vi "数据主动和反控发送.vi"   [LabVIEW 2016, in "数据传输系统.lvlib"]
uses:
  <vilib>/ptbypt/NI_PtbyPt.lvlib
types:
  T1 = enum16{"00点", "01点", "02点", "03点", "04点", "05点", "06点", "07点", "08点", "09点", "10点", "11点", "12点", "13点", "14点", "15点", "16点", "17点", "18点", "19点", "20点", "21点", "22点", "23点"}
  T2 = enum16{"关闭", "星期日", "星期一", "星期二", "星期三", "星期四", "星期五", "星期六"}
  T3 = typedef "LVDateTimeRec.ctl" = cluster{"秒数的小数部分":dbl, "秒":i32, "分":i32, "时":i32, "日":i32, "月":i32, "年":i32, "天数（周）":i32, "天数（年）":i32, "DST":i32}
  T4 = cluster{"CODMn":bool, "CODCr":bool, "DO":bool, "铜":bool, "PH":bool, "氨氮":bool, "比电导率":bool, "水温":bool, "盐度(海水)":bool, "浊度":bool, "总氮":bool, "总磷":bool, "叶绿素a":bool, "藻密度":bool, "水位":bool, "流速":bool, "瞬时流量":bool, "累积流量":bool}
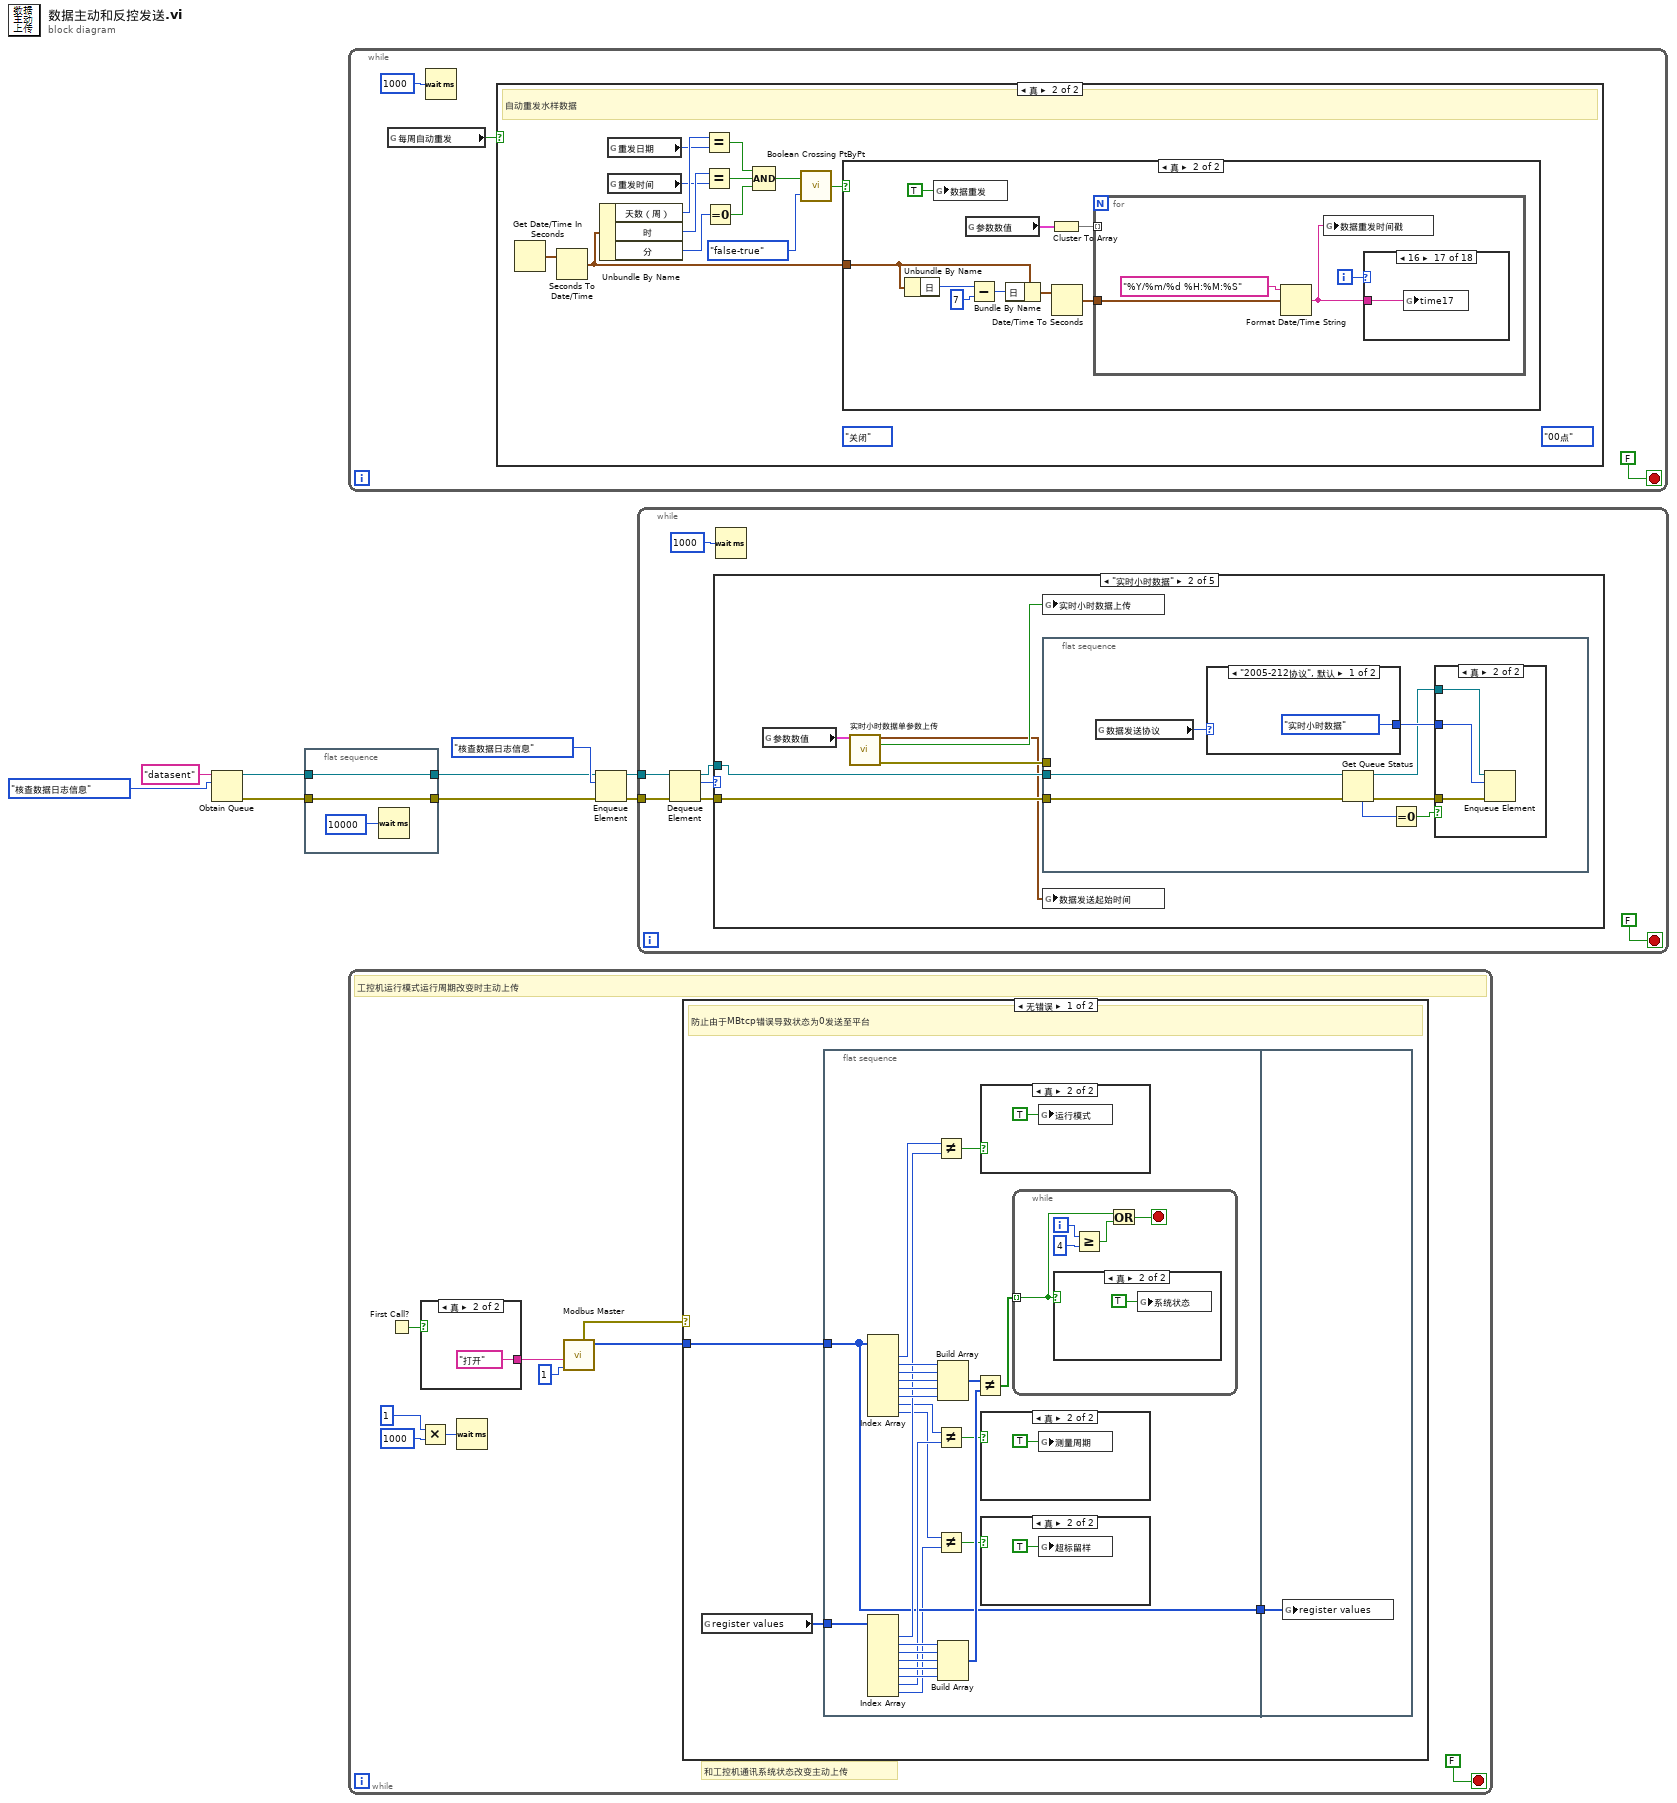
[diagram p0: block diagram]
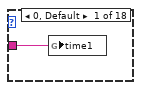
[diagram p4: hidden frame]
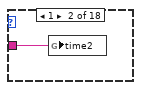
[diagram p5: hidden frame]
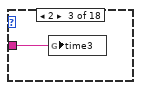
[diagram p6: hidden frame]
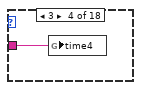
[diagram p7: hidden frame]
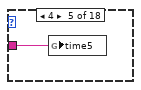
[diagram p8: hidden frame]
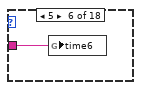
[diagram p9: hidden frame]
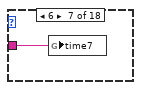
[diagram p10: hidden frame]
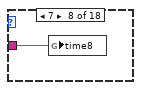
[diagram p11: hidden frame]
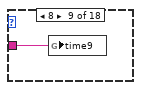
[diagram p12: hidden frame]
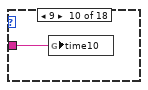
[diagram p13: hidden frame]
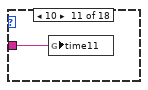
[diagram p14: hidden frame]
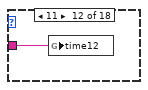
[diagram p15: hidden frame]
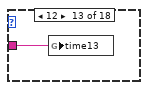
[diagram p16: hidden frame]
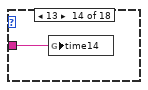
[diagram p17: hidden frame]
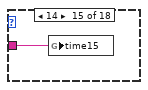
[diagram p18: hidden frame]
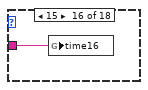
[diagram p19: hidden frame]
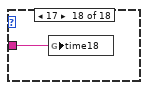
[diagram p20: hidden frame]
diagram:
  n1 = Obtain Queue(name (unnamed)="datasent" ("名称（未命名）"), element data type=enum16{"实时小时数据", "核查数据日志信息", "其他信息", "反控命令"}."核查数据日志信息") -> (queue out=w4:refnum<queue>, error out=w2:errorcluster)  [unwired: 3 in, 1 out]
  n2 = flat-sequence {
    tunnel: w4 -> [w11]
    tunnel: [w11] -> w3
    tunnel: w2 -> [w10]
    tunnel: [w10] -> w1
    frame #0 {
      n3 = Wait (ms)(milliseconds to wait=u32 10000 ("等待时间（毫秒）")) -> ()  [unwired: 1 out]
    }
  }
  n4 = while {
    stop <- FALSE stop-if-true
    n5 = global read "断电保存全局.vi" "每周自动重发"() -> (w14:bool)
    n6 = Wait (ms)(milliseconds to wait=u32 1000 ("等待时间（毫秒）")) -> ()  [unwired: 1 out]
    n7 = case shown="真" w14 {
      frame False {
      }
      frame True {
        (unwired) T1."00点"
        (unwired) T2."关闭"
        # "自动重发水样数据"
        n8 = Get Date/Time In Seconds() -> (seconds since 1Jan1904=w28:timestamp)
        n9 = Seconds To Date/Time(time stamp (now)=w28) -> (date time rec=w22:T3)  [unwired: 1 in]
        n10 = Unbundle By Name(w22) -> ("天数（周）"=w27:i32, "时"=w18:i32, "分"=w26:i32)
        n11 = global read "断电保存全局.vi" "重发日期"() -> (w17:T2)
        n12 = global read "断电保存全局.vi" "重发时间"() -> (w16:T1)
        n13 = Equal?(x=w27, y=w17) -> (x = y?=w25:bool)
        n14 = Equal?(x=w18, y=w16) -> (x = y?=w24:bool)
        n15 = Equal To 0?(x=w26) -> (x = 0?=w23:bool)
        n16 = Compound Arithmetic op=AND ("复合运算")(w25, w24, w23) -> (w21:bool)
        n17 = call <vilib>:"Boolean Crossing PtByPt.vi"("direction"=enum16{"either", "false-true", "true-false"}."false-true", "input"=w21) -> ("crossing"=w20:bool)  [unwired: 1 in]
        n18 = case shown="真" w20 {
          tunnel: w22 -> [_ w32]
          frame False {
          }
          frame True {
            n19 = Unbundle By Name(w32) -> ("日"=w35:i32)
            n20 = global write "断电保存全局.vi" "数据重发"(TRUE ("数据重发")) -> ()
            n21 = global read "全局1.vi" "参数数值"() -> (w30:T4)
            n22 = Subtract(x=w35, y=7) -> (x-y=w33:i32)
            n23 = Bundle By Name(cluster=w32, "日"=w33) -> (w36:T3)
            n24 = Cluster To Array(cluster=w30) -> (array=w37:bool[])
            n25 = Date/Time To Seconds(2:w36) -> (0:w31:timestamp)  [unwired: 1 in]
            n26 = for {
              tunnel: w37 -> [_] mode=indexing
              tunnel: w31 -> [w39]
              i -> [w40]
              n27 = Format Date/Time String(time format string (%c)="%Y/%m/%d %H:%M:%S" ("时间格式字符串(%c)"), seconds (now)=w39) -> (date/time string=w38:string)  [unwired: 1 in]
              n28 = global write "断电保存全局.vi" "数据重发时间戳"(w38) -> ()
              n29 = case shown="16" w40 {
                tunnel: w38 -> [w42 w43 w44 w45 w46 w47 w48 w49 w50 w51 w52 w53 w54 w55 w56 w57 w58 w59]
                frame 0, Default {
                  n30 = global write "全局 水样时间.vi" "time1"(w42) -> ()
                }
                frame 1 {
                  n31 = global write "全局 水样时间.vi" "time2"(w43) -> ()
                }
                frame 2 {
                  n32 = global write "全局 水样时间.vi" "time3"(w44) -> ()
                }
                frame 3 {
                  n33 = global write "全局 水样时间.vi" "time4"(w45) -> ()
                }
                frame 4 {
                  n34 = global write "全局 水样时间.vi" "time5"(w46) -> ()
                }
                frame 5 {
                  n35 = global write "全局 水样时间.vi" "time6"(w47) -> ()
                }
                frame 6 {
                  n36 = global write "全局 水样时间.vi" "time7"(w48) -> ()
                }
                frame 7 {
                  n37 = global write "全局 水样时间.vi" "time8"(w49) -> ()
                }
                frame 8 {
                  n38 = global write "全局 水样时间.vi" "time9"(w50) -> ()
                }
                frame 9 {
                  n39 = global write "全局 水样时间.vi" "time10"(w51) -> ()
                }
                frame 10 {
                  n40 = global write "全局 水样时间.vi" "time11"(w52) -> ()
                }
                frame 11 {
                  n41 = global write "全局 水样时间.vi" "time12"(w53) -> ()
                }
                frame 12 {
                  n42 = global write "全局 水样时间.vi" "time13"(w54) -> ()
                }
                frame 13 {
                  n43 = global write "全局 水样时间.vi" "time14"(w55) -> ()
                }
                frame 14 {
                  n44 = global write "全局 水样时间.vi" "time15"(w56) -> ()
                }
                frame 15 {
                  n45 = global write "全局 水样时间.vi" "time16"(w57) -> ()
                }
                frame 16 {
                  n46 = global write "全局 水样时间.vi" "time17"(w58) -> ()
                }
                frame 17 {
                  n47 = global write "全局 水样时间.vi" "time18"(w59) -> ()
                }
              }
            }
          }
        }
      }
    }
  }
  n48 = while {
    stop <- FALSE stop-if-true
    # "和工控机通讯系统状态改变主动上传"
    # "工控机运行模式运行周期改变时主动上传"
    n49 = First Call?() -> (First Call?: T/F=w60:bool)
    n50 = Multiply(x=u32 1, y=u32 1000 ("等待时间（毫秒）")) -> (x*y=w67:u32)
    n51 = case shown="真" w60 {
      tunnel: ["读取" ("读取写入选择") "打开" ("读取写入选择")] -> w64
      frame False {
      }
      frame True {
      }
    }
    n52 = Wait (ms)(milliseconds to wait=w67) -> ()  [unwired: 1 out]
    n53 = call "Modbus Master.vi"("Unit ID"=u8 1, "读取写入选择"=w64) -> ("register values"=w62:u16[], "error out"=w61:errorcluster)  [unwired: 8 in]
    n54 = case shown="无错误" w61 {
      tunnel: w62 -> [w70 _]
      frame No Error {
        # "防止由于MBtcp错误导致状态为0发送至平台"
        n55 = global read "全局1.vi" "register values"() -> (w69:u16[])
        n56 = flat-sequence {
          tunnel: w70 -> [w75]
          tunnel: w69 -> [w95]
          tunnel: [w75] -> w71
          tunnel: w71 -> [w105]
          frame #0 {
            n57 = Index Array(array=w75) -> (element #1=w82:u16, element #2=w94:u16, element #3=w93:u16, element #4=w92:u16, element #5=w91:u16, element #6=w90:u16, element #7=w80:u16, element #8=w74:u16)  [unwired: 8 in]
            n58 = Index Array(array=w95) -> (element #1=w81:u16, element #2=w89:u16, element #3=w88:u16, element #4=w87:u16, element #5=w86:u16, element #6=w85:u16, element #7=w79:u16, element #8=w73:u16)  [unwired: 8 in]
            n59 = Not Equal?(x=w82, y=w81) -> (x != y?=w77:bool)
            n60 = Not Equal?(x=w80, y=w79) -> (x != y?=w78:bool)
            n61 = Not Equal?(x=w74, y=w73) -> (x != y?=w72:bool)
            n62 = Build Array(w94, w93, w92, w91, w90) -> (w84:u16[])
            n63 = Build Array(w89, w88, w87, w86, w85) -> (w83:u16[])
            n64 = Not Equal?(x=w84, y=w83) -> (x != y?=w76:bool[])
            n65 = case shown="真" w77 {
              frame False {
              }
              frame True {
                n66 = global write "全局1.vi" "运行模式"(TRUE) -> ()
              }
            }
            n67 = case shown="真" w78 {
              frame False {
              }
              frame True {
                n68 = global write "全局1.vi" "测量周期"(TRUE ("系统状态改变")) -> ()
              }
            }
            n69 = case shown="真" w72 {
              frame False {
              }
              frame True {
                n70 = global write "全局1.vi" "超标留样"(TRUE ("系统状态改变")) -> ()
              }
            }
            n71 = while {
              tunnel: w76 -> [w99] mode=indexing
              i -> [w101]
              stop <- w97 stop-if-true
              n72 = case shown="真" w99 {
                frame False {
                }
                frame True {
                  n73 = global write "全局1.vi" "系统状态"(TRUE ("系统状态改变")) -> ()
                }
              }
              n74 = Greater Or Equal?(x=w101, y=4) -> (x >= y?=w98:bool)
              n75 = Or(x=w99, y=w98) -> (x .or. y?=w97:bool)
            }
          }
          frame #1 {
            n76 = global write "全局1.vi" "register values"(w105) -> ()
          }
        }
      }
      frame Error {
      }
    }
  }
  n77 = Enqueue Element(queue=w3, element=enum16{"实时小时数据", "核查数据日志信息", "其他信息", "反控命令"}."核查数据日志信息", error in (no error)=w1) -> (queue out=w6:refnum<queue>, error out=w5:errorcluster)  [unwired: 1 in, 1 out]
  n78 = while {
    tunnel: w6 -> [w112]
    tunnel: w5 -> [w111]
    stop <- FALSE stop-if-true
    n79 = Dequeue Element(queue=w112, error in (no error)=w111) -> (queue out=w109:refnum<queue>, element=w110:enum16{"实时小时数据", "核查数据日志信息", "其他信息", "反控命令"}, error out=w108:errorcluster)  [unwired: 1 in, 1 out]
    n80 = case shown="\"实时小时数据\"" w110 {
      tunnel: w109 -> [_ w118 w136 _ w142]
      tunnel: w108 -> [_ w117 w135 _ w141]
      frame Default {
      }
      frame "实时小时数据" {
        n81 = global read "全局1.vi" "参数数值"() -> (w120:T4)
        n82 = call "实时小时数据单参数上传.vi"("参数数值"=w120) -> ("数据发送起始时间"=w115:timestamp, "实时小时数据上传"=w116:bool, "error out"=w119:errorcluster)  [unwired: 12 in]
        n83 = global write "全局1.vi" "实时小时数据上传"(w116) -> ()
        n84 = flat-sequence {
          tunnel: w119 -> [_]
          tunnel: w118 -> [w125]
          tunnel: w117 -> [w124]
          frame #0 {
            n85 = global read "断电保存全局.vi" "数据发送协议"() -> (w128:enum16{"2005-212协议", "2017-212协议"})
            n86 = case shown="\"2005-212协议\", 默认" w128 {
              tunnel: [enum16{"实时小时数据", "核查数据日志信息", "其他信息", "反控命令"}."实时小时数据" enum16{"实时小时数据", "核查数据日志信息", "其他信息", "反控命令"}."核查数据日志信息"] -> w127
              frame "2005-212协议", Default {
              }
              frame "2017-212协议" {
              }
            }
            n87 = Get Queue Status(queue=w125, error in (no error)=w124) -> (queue out=w122:refnum<queue>, error out=w121:errorcluster, # elements in queue=w126:i32)  [unwired: 1 in, 5 out]
            n88 = Equal To 0?(x=w126) -> (x = 0?=w123:bool)
            n89 = case shown="真" w123 {
              tunnel: w127 -> [_ w131]
              tunnel: w122 -> [_ w130]
              tunnel: w121 -> [_ w129]
              frame False {
              }
              frame True {
                n90 = Enqueue Element(queue=w130, element=w131, error in (no error)=w129) -> ()  [unwired: 1 in, 3 out]
              }
            }
          }
        }
        n91 = global write "全局1.vi" "数据发送起始时间"(w115) -> ()
      }
      frame "核查数据日志信息" {
        n92 = call "核查数据和日志信息出发送队列 (子VI).vi"() -> ("错误输出"=w137:errorcluster, "核查数据上传"=w134:bool)  [unwired: 10 in]
        n93 = global write "全局1.vi" "核查数据上传"(w134) -> ()
        n94 = flat-sequence {
          tunnel: w137 -> [_]
          tunnel: w136 -> [w140]
          tunnel: w135 -> [w139]
          frame #0 {
            n95 = Enqueue Element(queue=w140, element=enum16{"实时小时数据", "核查数据日志信息", "其他信息", "反控命令"}."实时小时数据", error in (no error)=w139) -> ()  [unwired: 1 in, 3 out]
          }
        }
      }
      frame "其他信息" {
      }
      frame "反控命令" {
        n96 = flat-sequence {
          tunnel: w142 -> [w147]
          tunnel: w141 -> [w145]
          frame #0 {
            n97 = global read "全局1.vi" "命令编码CN"() -> (w144:string)
            n98 = global read "全局1.vi" "数据"() -> (w143:string)
            n99 = call "读取反控数据解析(子VI).vi"("数据"=w143, "命令编码CN"=w144) -> ()  [unwired: 8 in, 2 out]
          }
          frame #1 {
            n100 = call "反控数据上传(子VI).vi"() -> ()  [unwired: 12 in]
          }
          frame #2 {
            n101 = Enqueue Element(queue=w147, element=enum16{"实时小时数据", "核查数据日志信息", "其他信息", "反控命令"}."实时小时数据", error in (no error)=w145) -> ()  [unwired: 1 in, 3 out]
          }
        }
      }
    }
    n102 = Wait (ms)(milliseconds to wait=u32 1000 ("等待时间（毫秒）")) -> ()  [unwired: 1 out]
  }
